vi "UserDefinedPath.vi"() -> (3 "ProDefPath":T1)   [LabVIEW 2017]
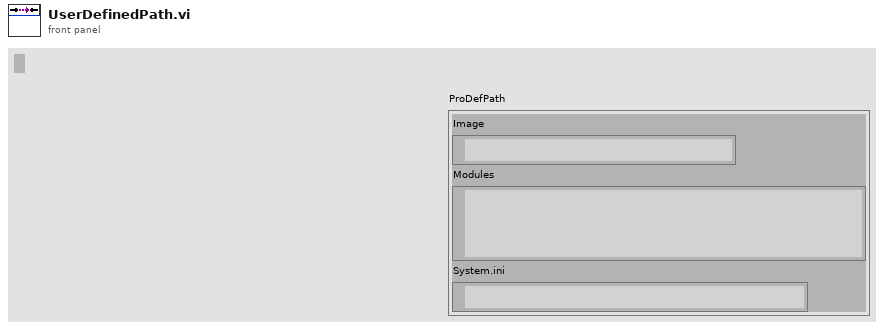
[diagram p1: front panel]
types:
  T1 = cluster{"Image":path, "Modules":path, "System.ini":path}
  T2 = enum32{"invalid app kind", "Development System", "Run Time System", "Student Edition", "Embedded LabVIEW", "Evaluation", "Custom"}
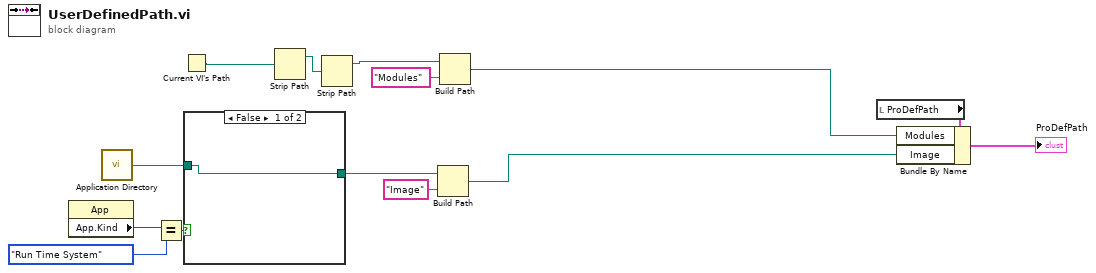
[diagram p0: block diagram]
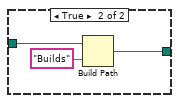
[diagram p2: hidden frame]
diagram:
  n1 = property class="App"() -> ("App.Kind"=w11:T2)  [unwired: 2 in, 2 out]
  n2 = call <vilib>:"Application Directory.vi"() -> ("Application Directory"=w14:path)
  n3 = Equal?(x=w11, y=T2."Run Time System") -> (x = y?=w9:bool)
  n4 = Current VI's Path() -> (path=w2:path)
  n5 = case shown="False" w9 {
    tunnel: w14 -> [w15 w18]
    tunnel: [w15 w16] -> w3
    frame False {
    }
    frame True {
      n6 = Build Path(base path=w18, name or relative path="Builds" ("名称或相对路径")) -> (appended path=w16:path)
    }
  }
  n7 = Strip Path(path=w2) -> (stripped path=w7:path)  [unwired: 1 out]
  n8 = Strip Path(path=w7) -> (stripped path=w5:path)  [unwired: 1 out]
  n9 = Build Path(base path=w3, name or relative path="Image" ("名称或相对路径")) -> (appended path=w1:path)
  n10 = Build Path(base path=w5, name or relative path="Modules" ("名称或相对路径")) -> (appended path=w4:path)
  n11 = local read "ProDefPath"() -> (w13:T1)
  n12 = Bundle By Name(cluster=w13, "Modules"=w4, "Image"=w1) -> (→"ProDefPath":T1)
